vi "CRIO write (SubVI).vi"(0 "Altitude Est":dbl, 6 "CO_NED":dbl[](array[numeric])=[0.0, 0.0], 7 "States":dbl[](array[numeric]), 8 "error IO":errorcluster, 9 "Array":u8[](array[numeric]), 10 "Port to Write (RT)":enum8{"1", "2", "3", "4"}(ring)=enum."3", 11 "FPGA VI Reference In":refnum<k20>) -> (4 "error out":errorcluster, 5 "FPGA VI Reference Out":refnum<k20>)   [LabVIEW 2014]
uses:
  <vilib>/Utility/error.llb/Error Cluster From Error Code.vi
  <vilib>/rvi/errors/niLvFpgaAdjustHostInterfaceError.vi
  <vilib>/rvi/interface/nirviReadWriteControl/nirviReadWriteControl.xnode
  FPGA Bitfiles/MinervaControlSy_FPGATarget_9870InterfaceDMA_4D1233B8.lvbitx
  cRIO/FPGA/9870 Interface DMA (FPGA).vi
  <vilib>/rvi/interface/nirviMethod/nirviMethod.xnode
  <vilib>/rvi/errors/niLvFpgaMergeErrorWithErrorCode.vi
  NiFpgaLv.dll
  <vilib>/FPGAPlugInAG/cRIO-9074/niLvFpga_WriteFifo_cRIO-9074.vi
panel:
  in  "Send pos":bool
  in  "d_offset":dbl
  out "Result":string
  # "10."
  # "20."
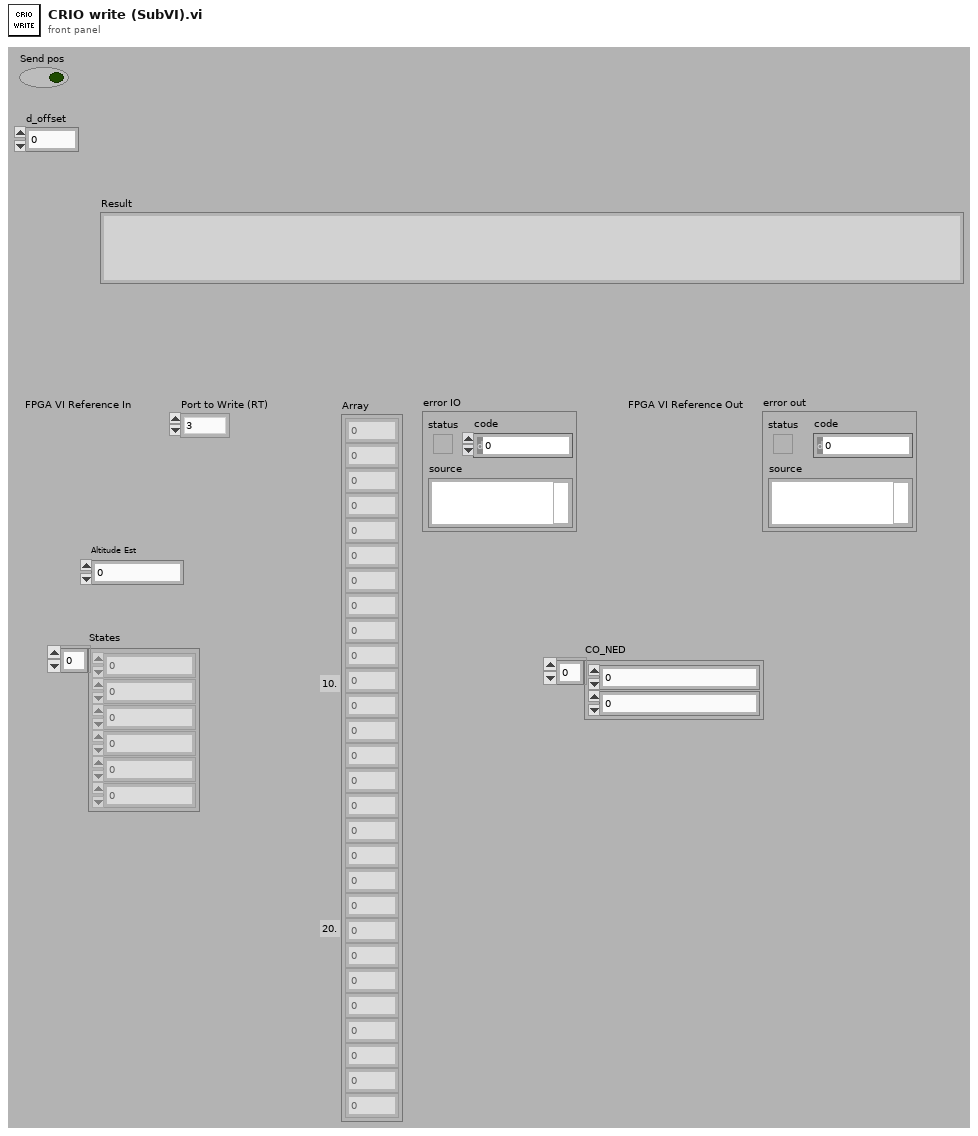
[diagram p1: front panel]
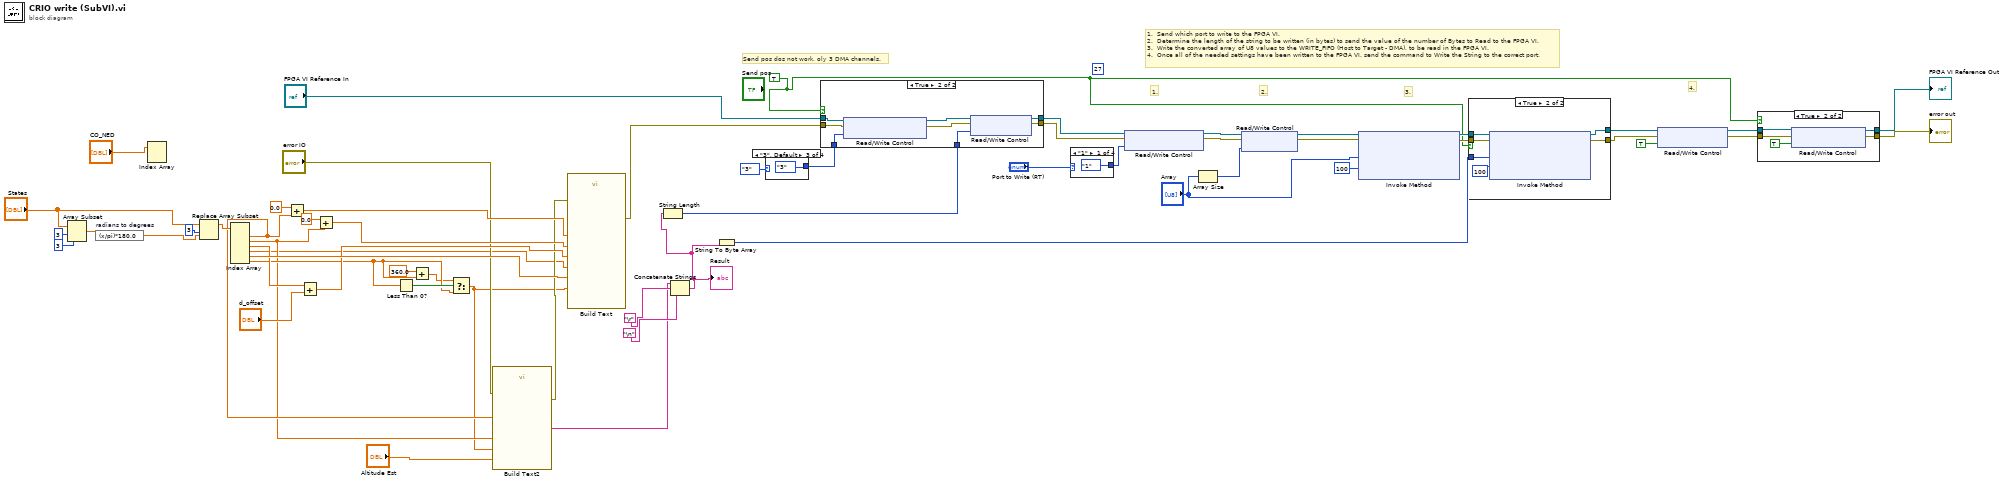
[diagram p0: block diagram]
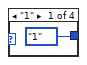
[diagram p5: hidden frame]
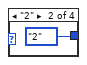
[diagram p6: hidden frame]
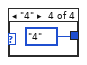
[diagram p7: hidden frame]
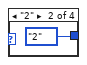
[diagram p8: hidden frame]
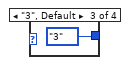
[diagram p9: hidden frame]
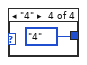
[diagram p10: hidden frame]
diagram:
  w12 = TRUE
  (unwired) 27 ("Timeout (ms)")
  # "Send pos dos not work, oly 3 DMA channels."
  # "1.  Send which port to write to the FPGA VI.\n2.  Determine the length of the string to be written (in bytes) to send the value of the number of Bytes to Read to the FPGA VI.\n3.  Write the converted array of U8 values to the WRITE_FIFO (Host to Target - DMA), to be read in the FPGA VI.\n4.  Once all of the needed settings have been written to the FPGA VI, send the command to Write the String to the correct port."
  # "4."
  # "3."
  # "2."
  # "1."
  n1 = Array Subset(array="States", index=3, length=3) -> (w29:dbl[])
  n2 = expression code="(x/pi)*180.0" "radians to degrees"(w29) -> (w26:dbl[])
  n3 = Index Array(array="CO_NED") -> ()  [unwired: 2 in, 2 out]
  n4 = Replace Array Subset(array="States", new element=w26, index=3) -> (w25:dbl[])
  n5 = Index Array(array=w25) -> (element #1=w4:dbl, element #2=w3:dbl, element #3=w23:dbl, element #4=w2:dbl, element #5=w46:dbl, element #6=w14:dbl)  [unwired: 6 in]
  n6 = Add(x=0.0, y=w4) -> (x+y=w20:dbl)
  n7 = Add(x=w23, y="d_offset") -> (x+y=w22:dbl)
  n8 = Add(x=0.0, y=w3) -> (x+y=w19:dbl)
  n9 = Less Than 0?(x=w14) -> (x < 0?=w16:bool)
  n10 = Add(x=360.0, y=w14) -> (x+y=w13:dbl)
  n11 = Select(t=w13, s=w16, f=w14) -> (s? t:f=w1:dbl)
  n12 = call "Build Text2"("alt"="Altitude Est", "N"=w4, "E"=w3, "psi"=w1, "error in (no error)"="error IO") -> ("Result"=w6:string, "error out"=w7:errorcluster)  [unwired: 9 in]
  n13 = call "Build Text"("phi"=w2, "psi"=w1, "N"=w20, "E"=w19, "D"=w22, "error in (no error)"=w7, "theta"=w46) -> ("error out"=w38:errorcluster)  [unwired: 7 in, 1 out]
  n14 = Concatenate Strings(w6, "\r", "\n") -> (w10:string)
  "Result" <- w10
  n15 = String Length(string=w10) -> (length=w42:i32)
  n16 = String To Byte Array(string=w10) -> (unsigned byte array=w40:u8[])
  n17 = case shown="\"3\", Default" enum8{"1", "2", "3", "4"}."3" ("Port to Write (RT)") {
    tunnel: [enum8{"0", "1", "2", "3", "4"}."1" ("Port To Write (FPGA)") enum8{"0", "1", "2", "3", "4"}."2" ("Port To Write (FPGA)") enum8{"0", "1", "2", "3", "4"}."3" ("Port To Write (FPGA)") enum8{"0", "1", "2", "3", "4"}."4" ("Port To Write (FPGA)")] -> w37
    frame "1" {
    }
    frame "2" {
    }
    frame "3", Default {
    }
    frame "4" {
    }
  }
  n18 = case shown="True" w12 {
    tunnel: [w64 w72] -> w48
    tunnel: [w63 w71] -> w47
    tunnel: w42 -> [_ w70]
    tunnel: "FPGA VI Reference In" -> [w64 w69]
    tunnel: w38 -> [w63 w67]
    tunnel: w37 -> [_ w65]
    frame False {
    }
    frame True {
      n19 = xnode "Read/Write Control"("FPGA VI Reference In"=w69, "error in"=w67, "Port To Write (FPGA2)"=w65) -> ("FPGA VI Reference Out"=w68:refnum<k20>, "error out"=w66:errorcluster)
      n20 = xnode "Read/Write Control"("FPGA VI Reference In"=w68, "error in"=w66, "Bytes to Send 2"=w70) -> ("FPGA VI Reference Out"=w72:refnum<k20>, "error out"=w71:errorcluster)
    }
  }
  n21 = case shown="\"1\"" "Port to Write (RT)" {
    tunnel: [enum8{"0", "1", "2", "3", "4"}."1" ("Port To Write (FPGA)") enum8{"0", "1", "2", "3", "4"}."2" ("Port To Write (FPGA)") enum8{"0", "1", "2", "3", "4"}."3" ("Port To Write (FPGA)") enum8{"0", "1", "2", "3", "4"}."4" ("Port To Write (FPGA)")] -> w58
    frame "1" {
    }
    frame "2" {
    }
    frame "3", Default {
    }
    frame "4" {
    }
  }
  n22 = xnode "Read/Write Control"("FPGA VI Reference In"=w48, "error in"=w47, "Port To Write (FPGA)"=w58) -> ("FPGA VI Reference Out"=w55:refnum<k20>, "error out"=w54:errorcluster)
  n23 = Array Size(array="Array") -> (size(s)=w41:i32)
  n24 = xnode "Read/Write Control"("FPGA VI Reference In"=w55, "error in"=w54, "Bytes to Send"=w41) -> ("FPGA VI Reference Out"=w11:refnum<k20>, "error out"=w56:errorcluster)
  n25 = xnode "Invoke Method"("FPGA VI Reference In"=w11, "error in"=w56, "Data"="Array", "Timeout (ms)"=100) -> ("FPGA VI Reference Out"=w50:refnum<k20>, "error out"=w51:errorcluster)  [unwired: 1 out]
  n26 = case shown="True" w12 {
    tunnel: w51 -> [w77 w84]
    tunnel: w50 -> [w78 w83]
    tunnel: [w78 w82] -> w9
    tunnel: [w77 w81] -> w49
    tunnel: w40 -> [_ w80]
    frame False {
    }
    frame True {
      n27 = xnode "Invoke Method"("FPGA VI Reference In"=w83, "error in"=w84, "Data"=w80, "Timeout (ms)"=100) -> ("FPGA VI Reference Out"=w82:refnum<k20>, "error out"=w81:errorcluster)  [unwired: 1 out]
    }
  }
  n28 = xnode "Read/Write Control"("FPGA VI Reference In"=w9, "error in"=w49, "Write Data (FPGA)"=TRUE) -> ("FPGA VI Reference Out"=w35:refnum<k20>, "error out"=w34:errorcluster)
  n29 = case shown="True" w12 {
    tunnel: w35 -> [w86 w90]
    tunnel: w34 -> [w85 w89]
    tunnel: [w85 w88] -> w33
    tunnel: [w86 w87] -> w32
    frame False {
    }
    frame True {
      n30 = xnode "Read/Write Control"("FPGA VI Reference In"=w90, "error in"=w89, "Write Data (FPGA2)"=TRUE ("Write Data (FPGA)")) -> ("FPGA VI Reference Out"=w87:refnum<k20>, "error out"=w88:errorcluster)
    }
  }
  "error out" <- w33
  "FPGA VI Reference Out" <- w32
